vi "UI_General Setting.vi"(8 "error in (no error)":errorcluster) -> (0 "error out":errorcluster)   [LabVIEW 2015, in "ConfigHelper.lvlib"]
uses:
  ConfigHelper.lvlib
  Control_UI_General Setting.ctl
  Control_UI_General Setting State.ctl
  <vilib>/addons/PointValueMap/controls/PointMap.ctl
  <vilib>/addons/PointValueMap/PointValueMap.lvlib
panel:
  in  "OK Button":bool
  in  "Cancel Button":bool
  in  "Scan Time Gap (s)":dbl
  in  "Export Folder Path":path
  in  "Trigger Level (V)":dbl
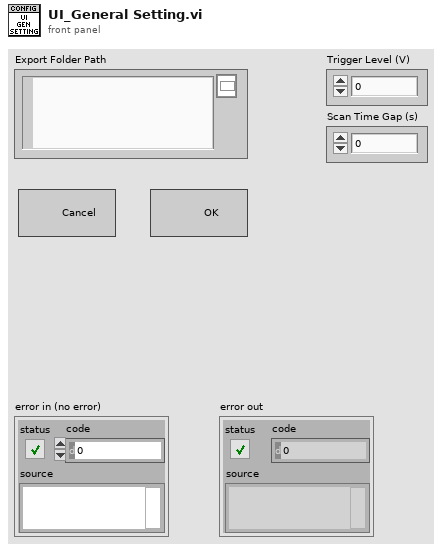
[diagram p1: front panel]
types:
  T1 = typedef "ConfigHelper.lvlib/Control_UI_General Setting.ctl" = cluster{"State":T2, "Map":T3, "Trigger Level":refnum<vi>, "Time Gap":refnum<vi>, "Path":refnum<vi>}
  T2 = typedef "ConfigHelper.lvlib/Control_UI_General Setting State.ctl" = enum16{"Init", "Read from PVM", "Wait", "Write to PVM", "Exit"}
  T3 = typedef "PointValueMap.lvlib/PointMap.ctl" = refnum<data-value>
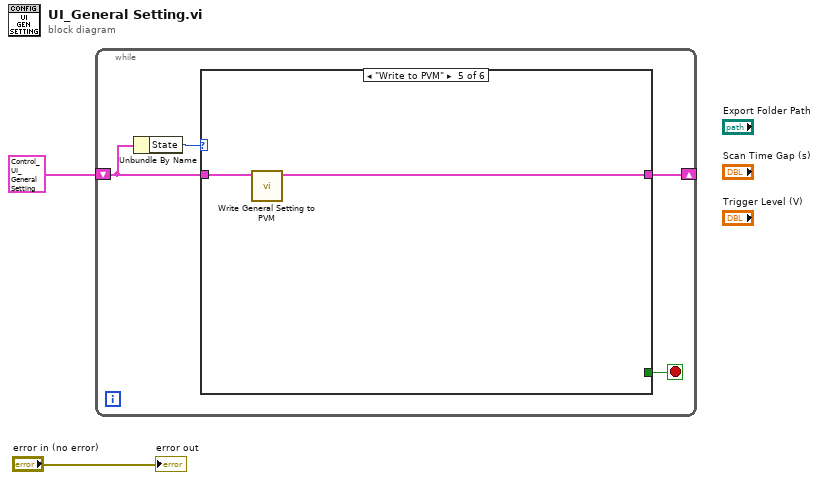
[diagram p0: block diagram]
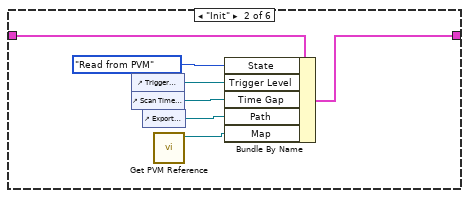
[diagram p3: hidden frame]
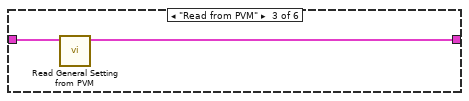
[diagram p4: hidden frame]
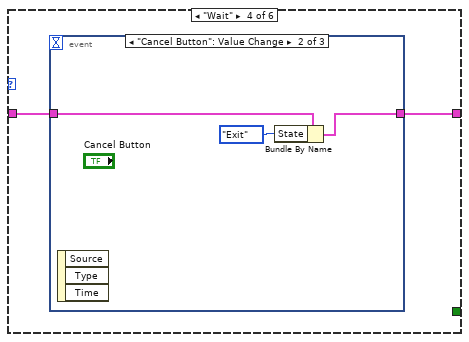
[diagram p5: hidden frame]
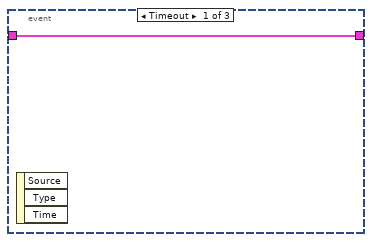
[diagram p6: hidden frame]
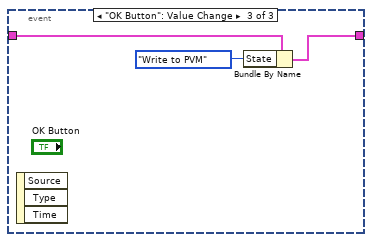
[diagram p7: hidden frame]
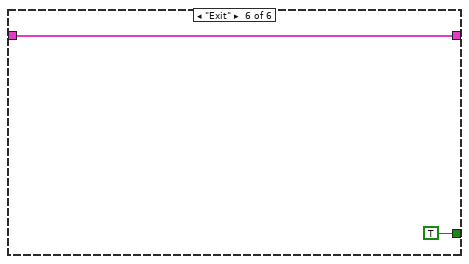
[diagram p8: hidden frame]
diagram:
  n1 = while {
    shift-right: [w4] -> _
    shift-left: T1 {"State"=enum."Init", "Map"=refnum, "Trigger Level"=refnum, "Time Gap"=refnum, "Path"=refnum} ("UI General Setting") -> [w5]
    stop <- w3 stop-if-true
    n2 = Unbundle By Name(w5) -> ("State"=w6:T2)
    n3 = case shown="\"Write to PVM\"" w6 {
      tunnel: w5 -> [w7 w10 w16 w18 w27 w29]
      tunnel: [w7 w9 w15 w17 w26 w29] -> w4
      tunnel: [_ _ _ _ _ TRUE] -> w3
      frame Default {
      }
      frame "Init" {
        n4 = control-ref of="Trigger Level (V)"() -> (w13:refnum<vi>)
        n5 = control-ref of="Scan Time Gap (s)"() -> (w12:refnum<vi>)
        n6 = control-ref of="Export Folder Path"() -> (w11:refnum<vi>)
        n7 = call "Get PVM Reference.vi"() -> ("Map Out"=w8:T3)  [unwired: 10 in, 1 out]
        n8 = Bundle By Name(cluster=w10, "State"=Control_UI_General_Setting_State."Read from PVM", "Trigger Level"=w13, "Time Gap"=w12, "Path"=w11, "Map"=w8) -> (w9:T1)
      }
      frame "Read from PVM" {
        n9 = call "Read General Setting from PVM.vi"("UI General Setting in"=w16) -> ("UI General Setting out"=w15:T1)  [unwired: 10 in]
      }
      frame "Wait" {
        n10 = event shown="[1] \"Cancel Button\": Value Change" {
          selector: _ -> [_ _ _]
          dyn-events: _ -> [_ _ _]
          timeout: _ -> [_ _ _]
          tunnel: w18 -> [w19 w22 w25]
          tunnel: [w19 w21 w24] -> w17
          event Timeout {
            n11 = event-data() -> ()  [unwired: 1 in, 3 out]
          }
          event "Cancel Button": Value Change {
            n12 = event-data() -> ()  [unwired: 1 in, 3 out]
            n13 = Bundle By Name(cluster=w22, "State"=Control_UI_General_Setting_State."Exit") -> (w21:T1)
          }
          event "OK Button": Value Change {
            n14 = event-data() -> ()  [unwired: 1 in, 3 out]
            n15 = Bundle By Name(cluster=w25, "State"=Control_UI_General_Setting_State."Write to PVM") -> (w24:T1)
          }
        }
      }
      frame "Write to PVM" {
        n16 = call "Write General Setting to PVM.vi"("UI General Setting in"=w27) -> ("UI General Setting out"=w26:T1)  [unwired: 10 in]
      }
      frame "Exit" {
      }
    }
  }
  "error out" <- "error in (no error)"
